vi "publish -- get -- 6.vi"(8 "request event":refnum<user-event>, 9 "response":refnum<user-event>) -> (2 "nnumber":dbl=1000.0 format="%#_10f")   [LabVIEW 2018]
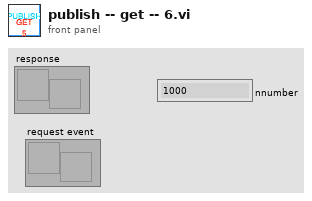
[diagram p1: front panel]
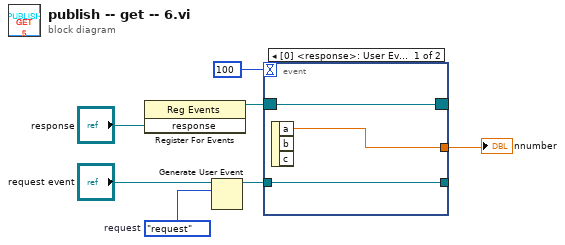
[diagram p0: block diagram]
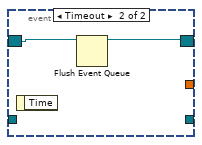
[diagram p2: hidden frame]
diagram:
  w7 = enum16{"request"}."request"  # request
  n1 = register-events("response") -> (reference out=w3:refnum<event-registration>)  [unwired: 2 in, 1 out]
  n2 = Generate User Event(user event="request event", event data cluster=w7) -> (user event out=w4:refnum<user-event>)  [unwired: 2 in, 1 out]
  n3 = event shown="[0] <response>: User Event" {
    selector: w3 -> [w8 w12]
    dyn-events: [w8 w11] -> _
    timeout: 100 -> [_ _]
    tunnel: [w10 _] -> w6
    tunnel: [w9 _] -> _
    tunnel: w4 -> [w9 _]
    event User Event {
      n4 = event-data() -> ("a"=w10:dbl)  [unwired: 1 in, 2 out]
    }
    event Timeout {
      n5 = event-data() -> ()  [unwired: 1 in, 1 out]
      n6 = Flush Event Queue(0:w12) -> (8:w11:refnum<event-registration>)  [unwired: 5 in, 2 out]
    }
  }
  "nnumber" <- w6
